vi "Sub_Variable_Length_Matrix.vi"(11 "Numeric":dbl) -> (3 "Array":dbl[][](array[numeric]))   [LabVIEW 2019]
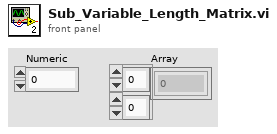
[diagram p1: front panel]
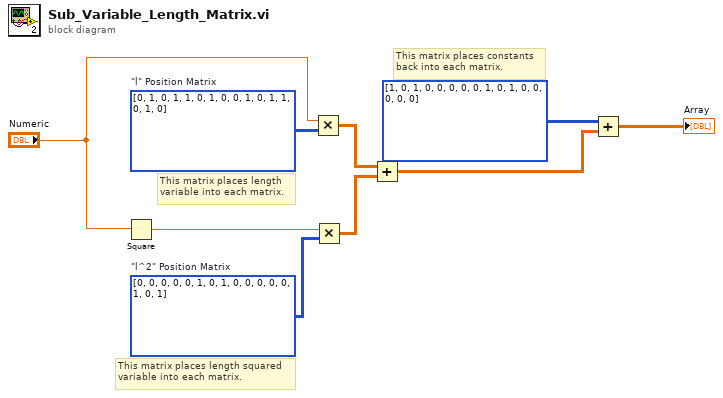
[diagram p0: block diagram]
diagram:
  w8 = i32[][] [[0, 0, 0, 0], [0, 1, 0, 1], [0, 0, 0, 0], [0, 1, 0, 1]]  # "l^2" Position Matrix
  w9 = i32[][] [[0, 1, 0, 1], [1, 0, 1, 0], [0, 1, 0, 1], [1, 0, 1, 0]]  # "l" Position Matrix
  # "This matrix places length squared\nvariable into each matrix."
  # "This matrix places length \nvariable into each matrix."
  # "This matrix places constants\nback into each matrix."
  n1 = Square(x="Numeric") -> (x^2=w6:dbl)
  n2 = Multiply(x="Numeric", y=w9) -> (x*y=w7:dbl[][])
  n3 = Multiply(x=w6, y=w8) -> (x*y=w5:dbl[][])
  n4 = Add(x=w7, y=w5) -> (x+y=w2:dbl[][])
  n5 = Add(x=i32[][] [[1, 0, 1, 0], [0, 0, 0, 0], [1, 0, 1, 0], [0, 0, 0, 0]], y=w2) -> (x+y=→"Array":dbl[][])
